vi "NanotecSMCPDDriver.get acceleration.vi"(0 "VISA resource name":refnum<visa-resource-name>, 1 "contollerID":i32=-1, 5 "error in (no error)":errorcluster) -> (14 "VISA resource name out":refnum<visa-resource-name>, 15 "contollerID out":i32=-1, 17 "acceleration [Hz/s]":dbl, 19 "error out":errorcluster)   [LabVIEW 2014, in "NanotecSMCPDDriver.lvlib"]
doc: "Gets the acceleration used for the trajectory of a movement."
uses:
  NanotecSMCPDDriver.lvlib
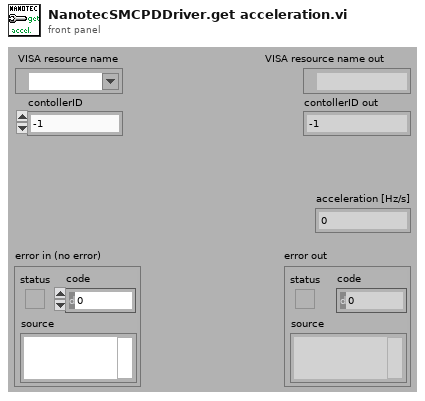
[diagram p1: front panel]
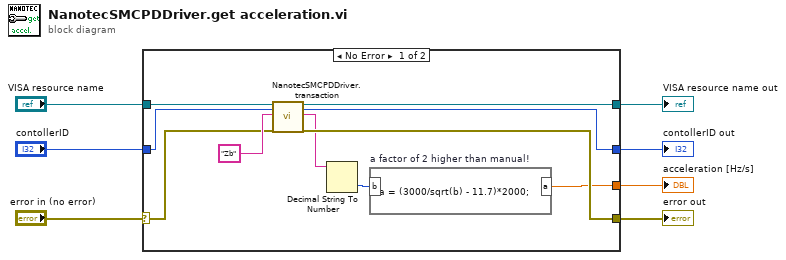
[diagram p0: block diagram]
diagram:
  n1 = case shown="No Error" "error in (no error)" {
    selector: "error in (no error)" -> [w10 w18]
    tunnel: [w16 w20] -> w7
    tunnel: [w15 w18] -> w6
    tunnel: "VISA resource name" -> [w12 w20]
    tunnel: "contollerID" -> [w11 w19]
    tunnel: [w17 w19] -> w3
    tunnel: [w8 _] -> w1
    frame No Error {
      n2 = call "NanotecSMCPDDriver.transaction.vi"("VISAresource"=w12, "contollerID"=w11, "commandString"="Zb", "error in (no error)"=w10) -> ("VISAresource out"=w16:refnum<visa-resource-name>, "contollerID out"=w17:i32, "response"=w13:string, "error out"=w15:errorcluster)  [unwired: 10 in, 2 out]
      n3 = Decimal String To Number(string=w13) -> (number=w9:i32)  [unwired: 2 in, 1 out]
      n4 = formula code="a = (3000/sqrt(b) - 11.7)*2000;" "a factor of 2 higher than manual!"("b"=w9) -> ("a"=w8:dbl)
    }
    frame Error {
    }
  }
  "acceleration [Hz/s]" <- w1
  "VISA resource name out" <- w7
  "error out" <- w6
  "contollerID out" <- w3
